vi "CC Convert RA and DEC to HHMMSS.vi"(11 "RA and DEC":T1) -> (0 "DEC String":string, 1 "RA String":string)   [LabVIEW 2024]
uses:
  typedefs/CC cluster RA and DEC.ctl
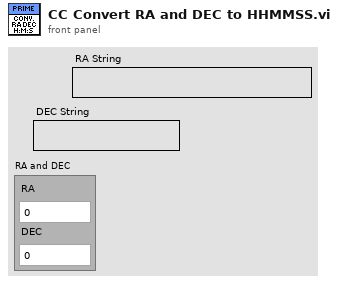
[diagram p1: front panel]
types:
  T1 = typedef "CC cluster RA and DEC.ctl" = cluster{"RA":dbl, "DEC":dbl}
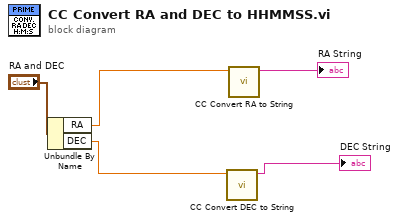
[diagram p0: block diagram]
diagram:
  n1 = Unbundle By Name("RA and DEC") -> ("RA"=w2:dbl, "DEC"=w4:dbl)
  n2 = call "CC Convert DEC to String.vi"("DEC"=w4) -> ("DEC String"=→"DEC String":string)  [unwired: 8 in, 2 out]
  n3 = call "CC Convert RA to String.vi"("RA"=w2) -> ("RA String"=→"RA String":string)  [unwired: 8 in, 2 out]
